vi "Event Actor.vi"(10 "Spawn":refnum<class "Spawn.lvclass">, 11 "Core Actor in":refnum<class "Core Actor.lvclass">) -> (0 "Error out":errorcluster, 3 "Core Actor out":refnum<class "Core Actor.lvclass">)   [LabVIEW 2025, in "jettl.lvlib" / "Actor.lvlib" / "Core Actor.lvclass"]
uses:
  Core Actor.lvclass
  Core Actor.lvclass/Core Actor.ctl
  Spawn/Spawn/Spawn.lvclass
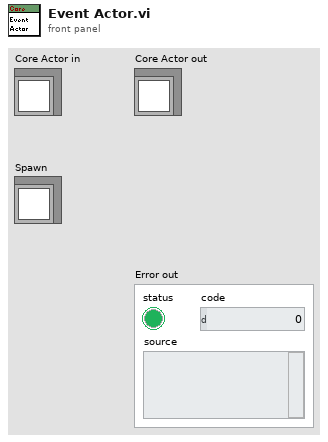
[diagram p1: front panel]
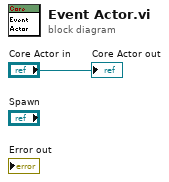
[diagram p0: block diagram]
diagram:
  "Core Actor out" <- "Core Actor in"
